vi "dataset.update_free.vi"(8 "error in":errorcluster, 11 "DatasetUpdateStaging in":refnum<class "DatasetUpdateStaging.lvclass">) -> (0 "error out":errorcluster, 3 "DatasetUpdateStaging out":refnum<class "DatasetUpdateStaging.lvclass">)   [LabVIEW 2020, in "DatasetUpdateStaging.lvclass"]
doc: "Releases the handle and its associated resources."
uses:
  DatasetUpdateStaging.lvclass
  DatasetUpdateStaging.lvclass/DatasetUpdateStaging.ctl
  client.lvlib
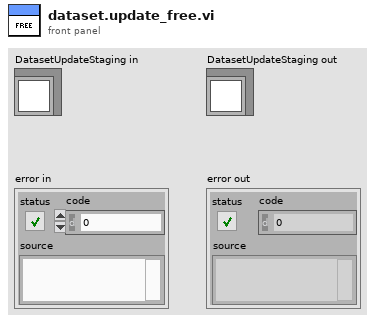
[diagram p1: front panel]
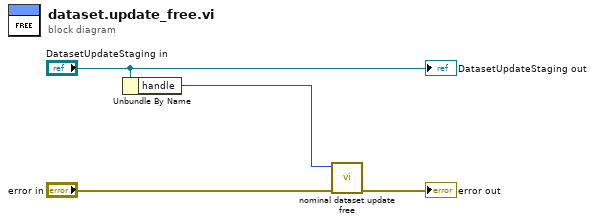
[diagram p0: block diagram]
diagram:
  n1 = Unbundle By Name("DatasetUpdateStaging in") -> ("handle"=w2:i32)
  n2 = call "nominal dataset update free.vi"("error in (no error)"="error in", "staging"=w2) -> ("error out"=→"error out":errorcluster)  [unwired: 8 in, 1 out]
  "DatasetUpdateStaging out" <- "DatasetUpdateStaging in"
